vi "Configure Modulation.vi"   [LabVIEW 2015, in "Agilent 3352X Series.lvlib"]
doc: "Allows users to configure different modulation settings on the function generator."
uses:
  <instrlib>/Agilent 3352X Series/Agilent 3352X Series.lvlib
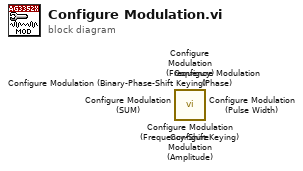
[diagram p0: block diagram]
diagram:
  n1 = call <instrlib>:"Configure Modulation (Frequency-Shift Keying).vi"() -> ()  [unwired: 14 in, 2 out]
  n2 = call <instrlib>:"Configure Modulation (Phase).vi"() -> ()  [unwired: 14 in, 2 out]
  n3 = call <instrlib>:"Configure Modulation (SUM).vi"() -> ()  [unwired: 14 in, 2 out]
  n4 = call <instrlib>:"Configure Modulation (Pulse Width).vi"() -> ()  [unwired: 14 in, 2 out]
  n5 = call <instrlib>:"Configure Modulation (Binary-Phase-Shift Keying).vi"() -> ()  [unwired: 14 in, 2 out]
  n6 = call <instrlib>:"Configure Modulation (Frequency).vi"() -> ()  [unwired: 14 in, 2 out]
  n7 = call <instrlib>:"Configure Modulation (Amplitude).vi"() -> ()  [unwired: 14 in, 2 out]
